vi "DraggingDresser.vi"() -> ()   [LabVIEW 2014]
panel:
  out "Force":dbl[](array[numeric])
  out "Angle for Minimum Force":i32 format="%.1f"
  in  "Coefficient of Kinetic Friction (Mu)":dbl format="%.1f"
  out "Waveform Graph":dbl[](graph)
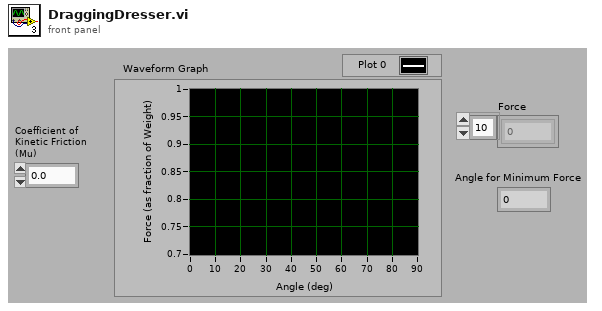
[diagram p1: front panel]
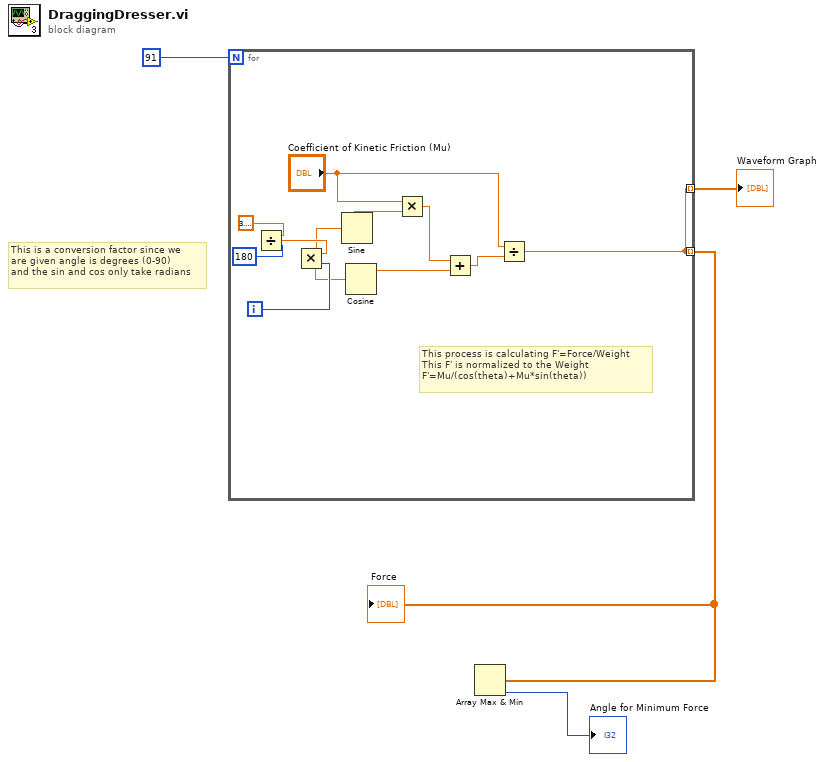
[diagram p0: block diagram]
diagram:
  # "This is a conversion factor since we\nare given angle is degrees (0-90) \nand the sin and cos only take radians"
  n1 = for {
    N: 91 -> [_]
    tunnel: [w10] -> w2 mode=indexing
    tunnel: [w10] -> w1 mode=indexing
    i -> [w9]
    # "This process is calculating F'=Force/Weight\nThis F' is normalized to the Weight\nF'=Mu/(cos(theta)+Mu*sin(theta))"
    n2 = Divide(x=3.141592653589793, y=180) -> (x/y=w8:dbl)
    n3 = Multiply(x=w8, y=w9) -> (x*y=w5:dbl)
    n4 = Sine(x=w5) -> (sin(x)=w15:dbl)
    n5 = Cosine(x=w5) -> (cos(x)=w13:dbl)
    n6 = Multiply(x="Coefficient of Kinetic Friction (Mu)", y=w15) -> (x*y=w14:dbl)
    n7 = Add(x=w14, y=w13) -> (x+y=w12:dbl)
    n8 = Divide(x="Coefficient of Kinetic Friction (Mu)", y=w12) -> (x/y=w10:dbl)
  }
  "Waveform Graph" <- w1
  "Force" <- w2
  n9 = Array Max & Min(array=w2) -> (min index (indices)=→"Angle for Minimum Force":i32)  [unwired: 3 out]
